vi "J1939 Conversion Lookup Table Initialize.vi"(8 "error in":errorcluster, 11 "scaling information":T1) -> (0 "error out":errorcluster {"code" min=0 max=0}, 3 "vi reference":T3)   [LabVIEW 2013, in "J1939.lvlib"]
uses:
  J1939.lvlib
  J1939 Conversion Lookup Table Reference.ctl
  API Types/Scaling Initialization.ctl
  CD/CD Conversion Lookup Table Parameters Cluster.ctl
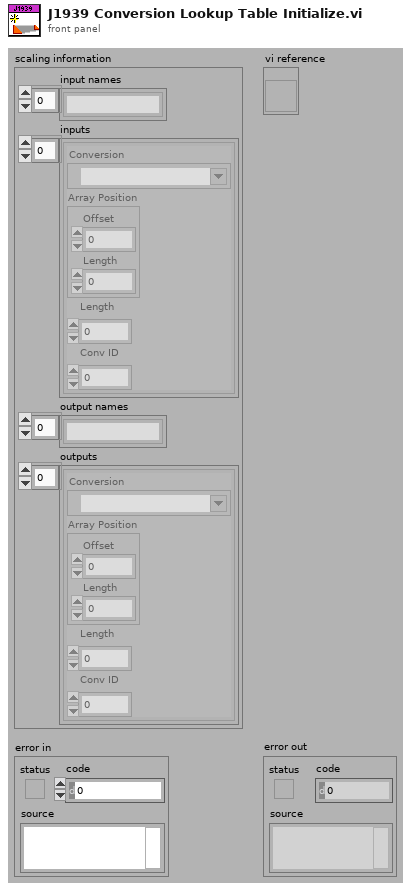
[diagram p1: front panel]
types:
  T1 = typedef "J1939.lvlib/scaling initialization.ctl" = cluster{"input names":string[], "inputs":T2[], "output names":string[], "outputs":T2[]}
  T2 = typedef "J1939.lvlib/CD Conversion Lookup Table Parameters Cluster.ctl" = cluster{"Conversion":refnum<k21>, "Array Position":cluster{"Offset":u32, "Length":u32}, "Length":u32, "Conv ID":u32}
  T3 = typedef "J1939.lvlib/J1939 Conversion Lookup Table Reference.ctl" = refnum<vi>
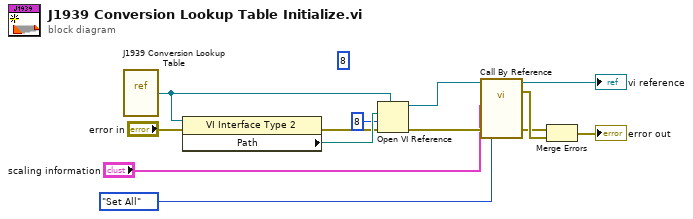
[diagram p0: block diagram]
diagram:
  (unwired) 8 ("options")
  n1 = vi-ref "J1939 Conversion Lookup Table.vi"() -> (w13:refnum<vi>)
  n2 = property class="VI Interface Type 2"(reference=w13, error in="error in") -> (error out=w10:errorcluster, "Path"=w12:path)  [unwired: 1 out]
  n3 = Open VI Reference(type specifier VI Refnum (for type only)=w13, vi path=w12, options=8, error in (no error)=w10) -> (vi reference=w9:refnum<vi>, error out=w4:errorcluster)  [unwired: 2 in]
  n4 = call-by-ref "?"(reference=w9, "command"=enum16{"Set All", "Lookup Parameters"}."Set All", "error in (no error)"=w4, "scaling information"="scaling information") -> (reference out=→"vi reference":refnum<vi>, error out=w8:errorcluster, 0:"error out"=w3:errorcluster)  [unwired: 7 in, 2 out]
  n5 = Merge Errors(w3, w8) -> (→"error out":errorcluster)
